vi "GPS Compute Target Bearing.vi"(9 "Current co-ordinates":T1={"Latitude"=2504.69148, "Longitude"=4361.44351} {"Longitude" format="%#_14g"; "Latitude" format="%#_14g"}, 10 "GPS Waypoint List Out":T1[](array[typedef])=[{"Latitude"=2504.67949, "Longitude"=4361.46974}] {"Longitude" format="%#_14g"; "Latitude" format="%#_14g"}) -> (3 "Target Bearing (degrees)":dbl)   [LabVIEW 2009]
uses:
  TypeDefs/Sensor Typedefs/GPS Data.ctl
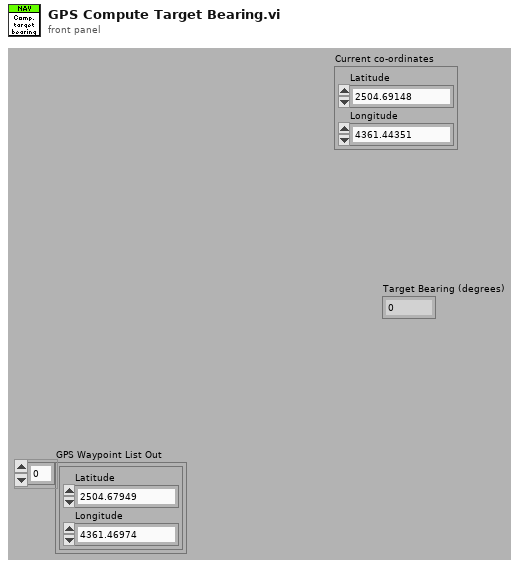
[diagram p1: front panel]
types:
  T1 = typedef "GPS Data.ctl" = cluster{"Latitude":dbl, "Longitude":dbl}
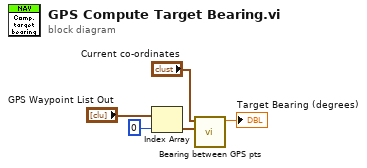
[diagram p0: block diagram]
diagram:
  n1 = Index Array(array="GPS Waypoint List Out", index=0) -> (element=w3:T1)
  n2 = call "Bearing between GPS pts.vi"("Pt.2"=w3, "Pt.1"="Current co-ordinates") -> ("Bearing Pt.1 to Pt.2"=→"Target Bearing (degrees)":dbl)  [unwired: 9 in]
